vi "ImagerForFlowbit5_com.vi"() -> ()   [LabVIEW 2011]
uses:
  <vilib>/Platform/TimedLoop/XDataNode/timing_clust.ctl
  <vilib>/Platform/TimedLoop/XDataNode/nitl_modes.ctl
  <vilib>/Platform/TimedLoop/XDataNode/wakeup.ctl
  <vilib>/Instr/_visa.llb/VISA Configure Serial Port (Instr).vi
  <vilib>/Utility/config.llb/Read Key (I32).vi
  <vilib>/Analysis/1siggen.llb/Riffle Array (I32).vi
  <vilib>/Platform/TimedLoop/XDataNode/XDataNode.xnode
  <vilib>/regexp/Match Regular Expression.xnode
  <vilib>/Analysis/NI_AALBase.lvlib
  <vilib>/vision/NI_Vision_Development_Module.lvlib
  <vilib>/Platform/TimedLoop/XDataNode/XDNodeRunTimeDep.lvlib
  <vilib>/Utility/config.llb/NI_LVConfig.lvlib
panel:
  out "frameNum":i32
  out "读取缓冲区 2":string
  out "返回数 2":u32
  out "Bounds.Right":i16
  out "停止循环":bool
  in  "Stimuli":i64=5
  in  "选项卡控件":enum32{"前面板", "参数设置", "OnLineMap"}(tab)
  out "Marker":bool
  out "log":string
  out "Stim_ID":i32(listbox)=1
  in  "开始/暂停":bool=TRUE
  in  "停止":bool
  out "重排的 Stim ID":i32[](array[numeric]) caption="重排的{X}"
  out "队列中元素数量":i32
  out "Image 2":T1(plugin-control)
  in  "热图":bool
  out "循环持续时间":i64
  out "Recording":bool
  out "grabLoop":i32
  out "writeing data":bool
  out "文件编号":u32
  out "address":i16=888 caption="地址" format="%.0x"
  in  "SaveParameter":bool
  in  "Pra_binType":enum16{"Extract", "Resample"}(ring)
  in  "Pra_FramesPerStim":i64=16000
  in  "Pra_Blk目录":path=path "C:/Expt/test"
  in  "Pra_TimeForPrepare(ms)":u32=1000
  in  "Pra_stim protocol":T2(array[ring])=[enum."recording data", enum."writing data"]
  in  "Pra_blank stim":u8
  in  "Pra_wait（ms）":u32=10
  in  "Pra_ISI（ms）":u32=8000
  in  "Pra_FrameBin":i32=25
  in  "Pra_datatype":u16(ring)=13 items=["U8"=11, "I16"=12, "U32"=13, "SGL"=14]
  in  "FrameWidth":i64=704
  in  "FrameHeight":i64=576
  in  "LoadParameter":bool
  in  "Pra_bin":enum16{"1*1", "2*2"}(ring)
  in  "maker":u32[](array[numeric])
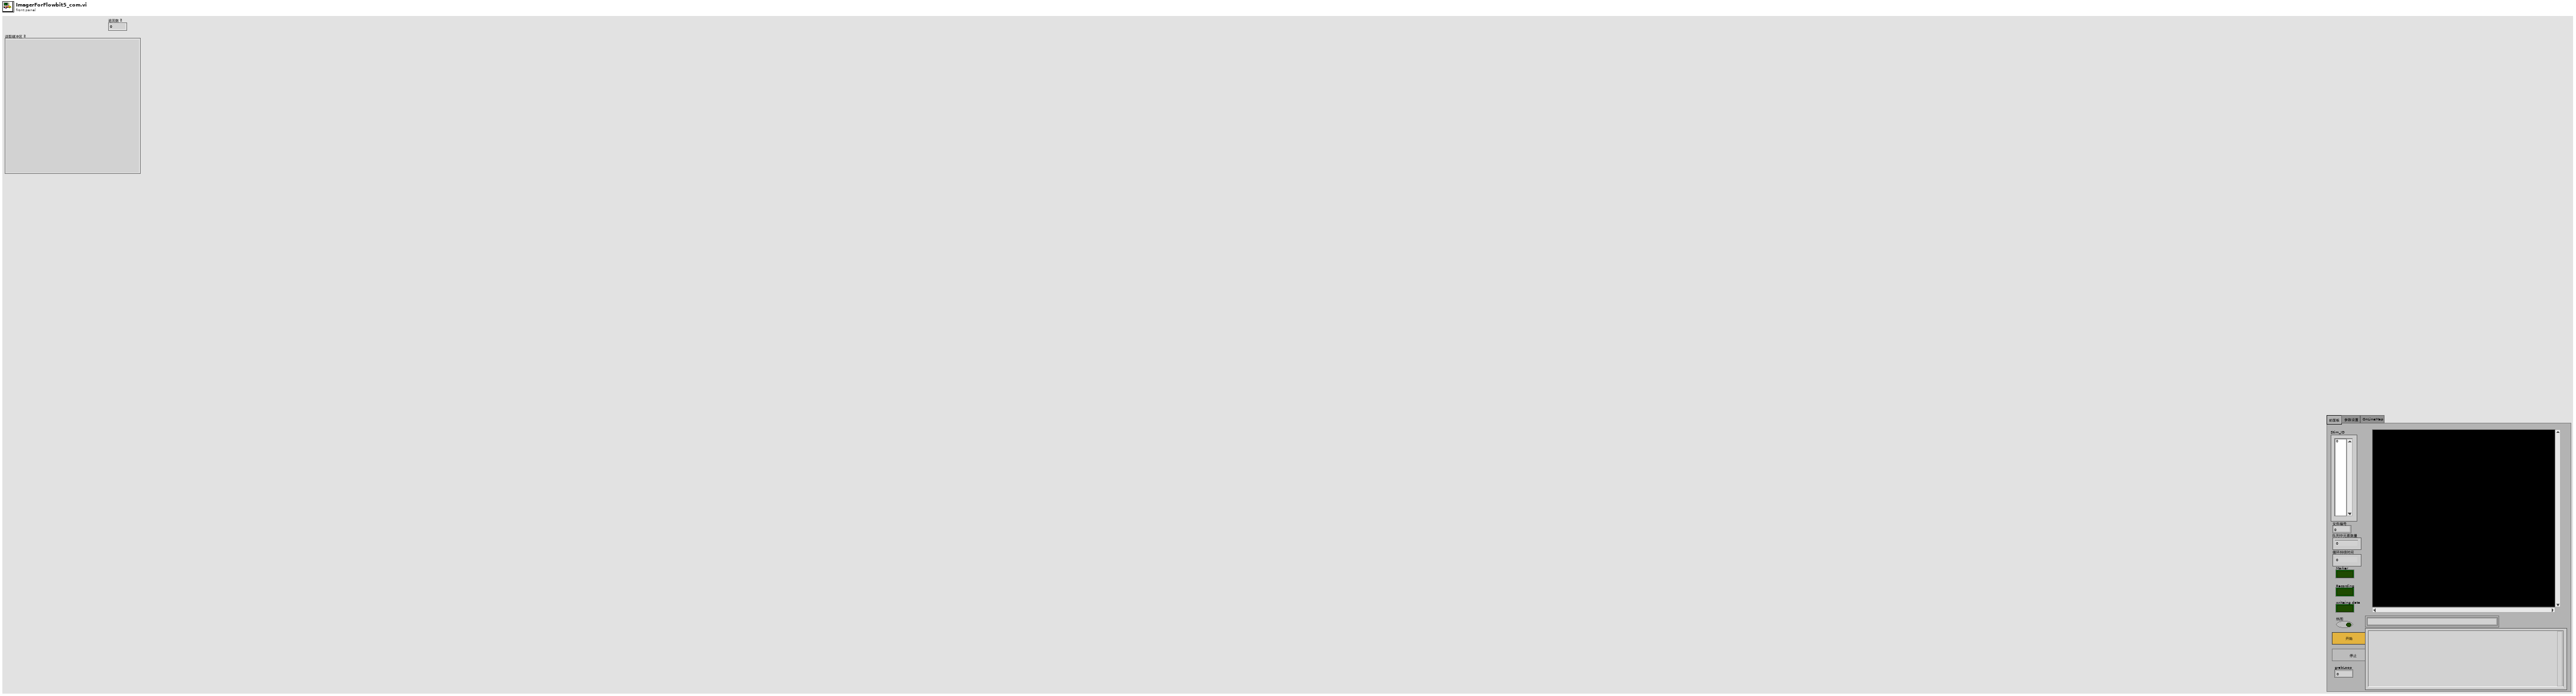
[diagram p1: front panel]
types:
  T1 = typedef "IMAQ Image.ctl" = refnum<image>
  T2 = enum16{"wait", "prep stim", "show stim", "wait respirator", "recording data", "Blank stim", "wait heart", "ISI", "DR/R", "wait calibrate", "openLightShutter", "closeLightShutter", "writing data"}[]
  T3 = typedef "Image Type" = u32
  T4 = enum16{"Disable External Trigger", "Enable External Trigger"}
  T5 = enum32{"Auto Detect", "RoadRunner", "Raven", "R64"}
  T6 = typedef "LVAllMonitorsDisplayTypeDef.ctl" = cluster{"Bounds":cluster{"Left":i16, "Top":i16, "Right":i16, "Bottom":i16}, "Depth":i16}[]
  T7 = cluster{"Bounds":cluster{"Left":i16, "Top":i16, "Right":i16, "Bottom":i16}, "Depth":i16}
  T8 = typedef "NI_LVConfig.lvlib/Config Data RefNum.ctl" = refnum<k1>
  T9 = enum16{"big-endian, network order", "native, host order", "little-endian"}
  T10 = enum16{"open", "replace", "create", "open or create", "replace or create", "replace or create with confirmation"}
  T11 = typedef "XDNodeRunTimeDep.lvlib/timing_clust.ctl" = cluster{"Expected End [f-1]":u64, "Actual End [f-1]":u64, "Finished Late? [f-1]":bool, "Expected End [i-1]":u64, "Actual End [i-1]":u64, "Finished Late? [i-1]":bool, "Expected Start [i]":u64, "Actual Start [i]":u64, "Expected Start [f]":u64, "Actual Start [f]":u64, "Source Name":string, "Structure Name":string, "Period":i64, "Deadline":i64, "Offset":i64, "Start":i64, "Priority":i32, "Timeout":i32, "Mode":T12, "Wakeup Reason":T13, "Error":errorcluster, "Source Type":string, "Secondary Source Type":string, "Global End Time":u64, "Global Start Time":u64, "Frame Duration":u64, "Iteration Duration":u64, "Assigned CPU":i32, "I/O Scan Engine Mode":u32}
  T12 = typedef "XDNodeRunTimeDep.lvlib/nitl_modes.ctl" = enum32{"No Change", "Process missed periods, maintain original phase", "Discard missed periods, maintain original phase", "Process missed periods, ignore original phase", "Discard missed periods, ignore original phase"}
  T13 = typedef "XDNodeRunTimeDep.lvlib/wakeup.ctl" = enum32{"Normal", "Aborted", "Asynchronous wakeup", "Timing source error", "Timed loop error", "Timeout"}
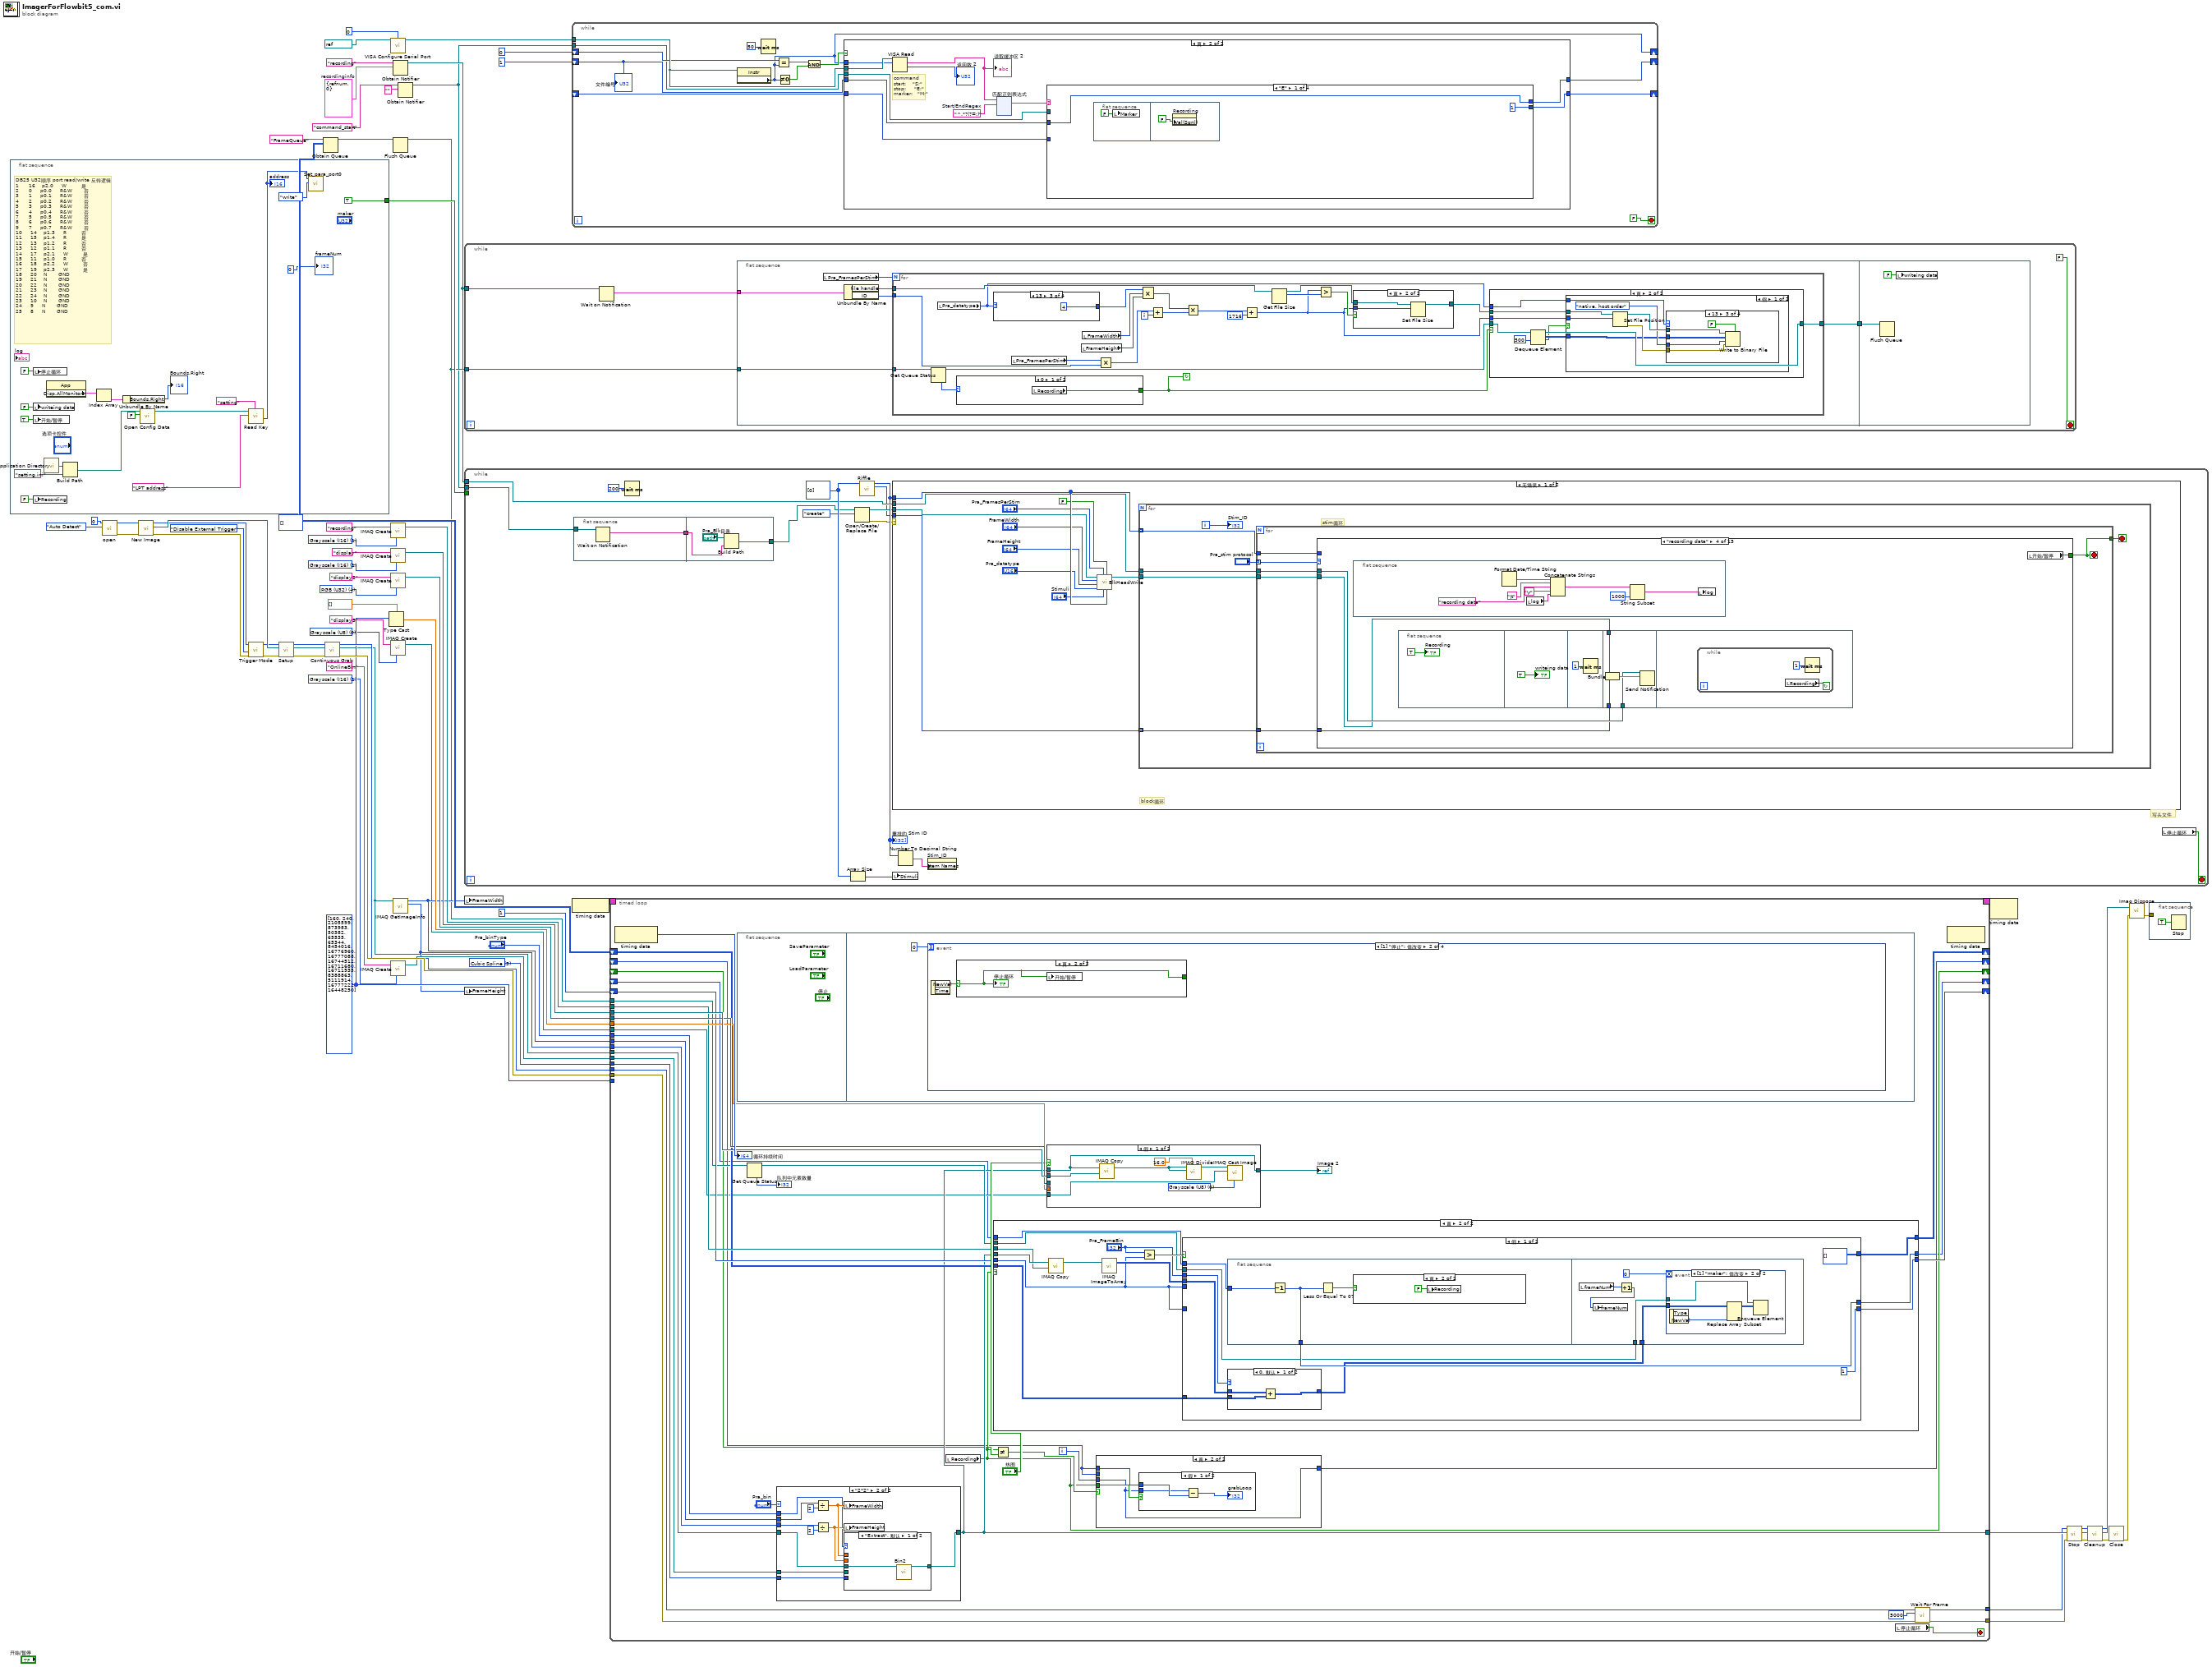
[diagram p0: block diagram]
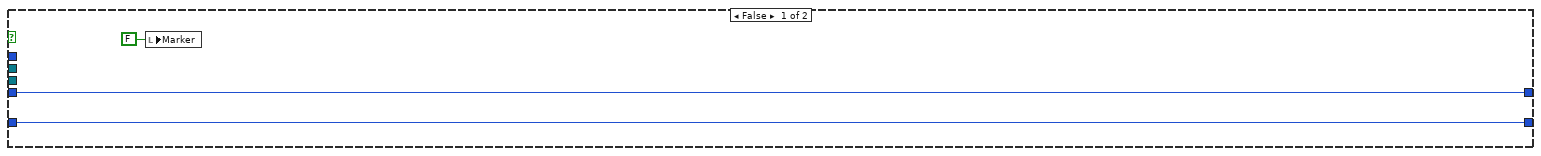
[diagram p2: hidden frame]
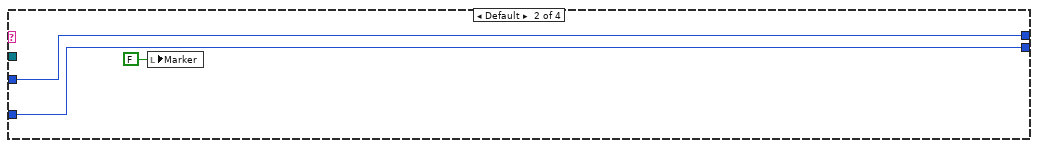
[diagram p3: hidden frame]
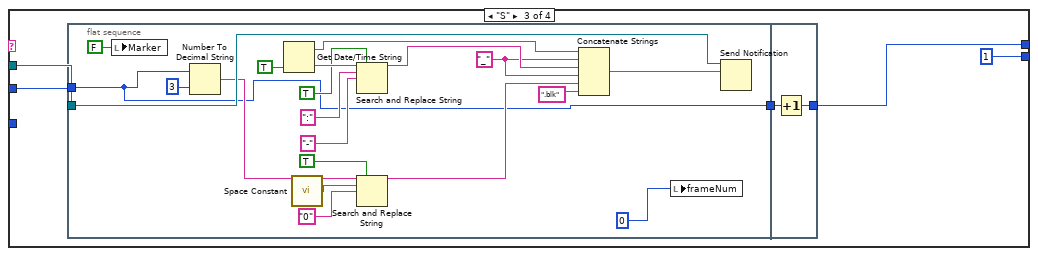
[diagram p4: hidden frame]
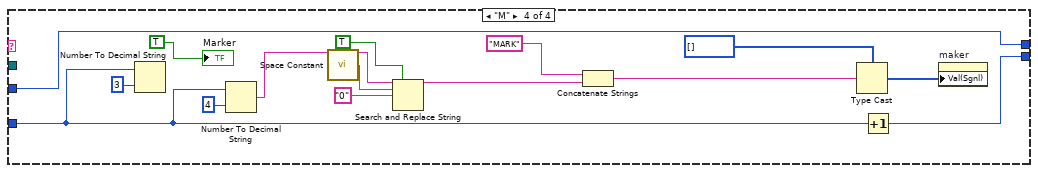
[diagram p5: hidden frame]
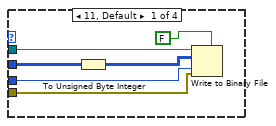
[diagram p7: hidden frame]
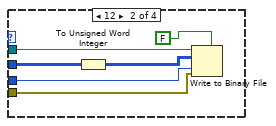
[diagram p8: hidden frame]
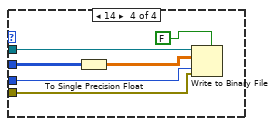
[diagram p9: hidden frame]
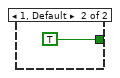
[diagram p11: hidden frame]
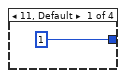
[diagram p13: hidden frame]
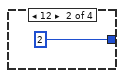
[diagram p14: hidden frame]
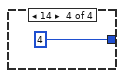
[diagram p15: hidden frame]
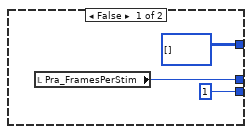
[diagram p16: hidden frame]
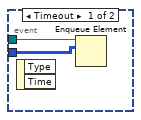
[diagram p18: hidden frame]
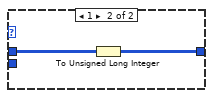
[diagram p19: hidden frame]
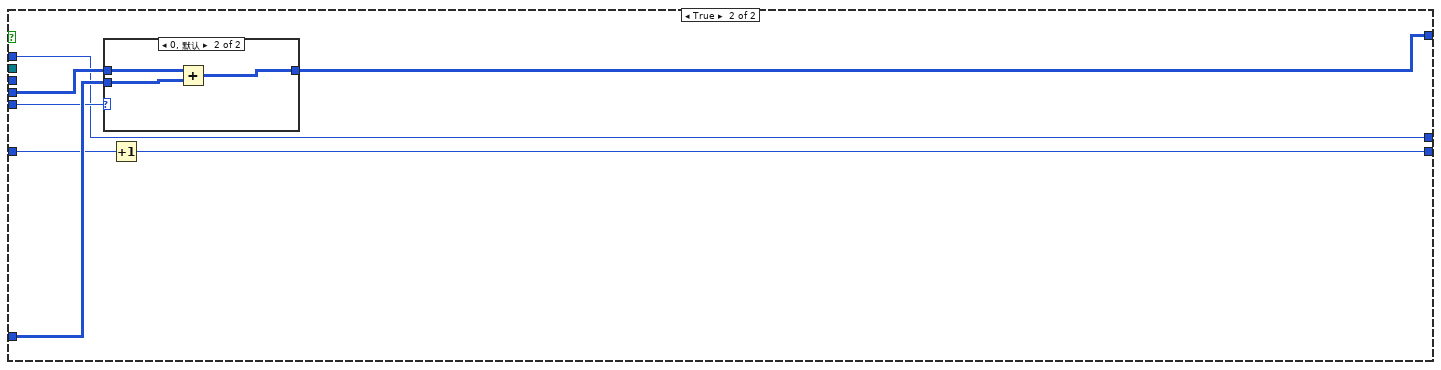
[diagram p20: hidden frame]
diagram:
  w10 = cluster{"file handle":refnum<file>, "ID":i32} {"file handle"=refnum, "ID"=0}  # recordinginfo
  w15 = T3 0 items=["Grayscale (U8)", "Grayscale (I16)", "Grayscale (SGL)", "Complex (CSG)", "RGB (U32)", "HSL (U32)", "RGB (U64)", "Grayscale (U16)"] ("Image Type")
  w20 = u32 3 items=["Zero Order", "Bi-Linear", "Quadratic", "Cubic Spline"] ("Interpolation Type")
  w22 = T3 1 items=["Grayscale (U8)", "Grayscale (I16)", "Grayscale (SGL)", "Complex (CSG)", "RGB (U32)", "HSL (U32)", "RGB (U64)", "Grayscale (U16)"] ("Image Type")
  w25 = u32[][] []
  w34 = T3 4 items=["Grayscale (U8)", "Grayscale (I16)", "Grayscale (SGL)", "Complex (CSG)", "RGB (U32)", "HSL (U32)", "RGB (U64)", "Grayscale (U16)"] ("Image Type")
  w32 = u32[] [160, 240, 2105599, 873983, 50382, 65535, 65344, 8454016, 16776960, 16777088, 16744512, 16711680, 16711935, 8388863, 5111914, 16777222, 16448250] ("数组")
  w38 = T3 1 items=["Grayscale (U8)", "Grayscale (I16)", "Grayscale (SGL)", "Complex (CSG)", "RGB (U32)", "HSL (U32)", "RGB (U64)", "Grayscale (U16)"] ("Image Type")
  w39 = T3 1 items=["Grayscale (U8)", "Grayscale (I16)", "Grayscale (SGL)", "Complex (CSG)", "RGB (U32)", "HSL (U32)", "RGB (U64)", "Grayscale (U16)"] ("Image Type")
  n1 = flat-sequence {
    tunnel: [TRUE ("Zoom to Fit Mode")] -> w27
    frame #0 {
      # "DB25\tU32顺序\tport\tread/write\t反转逻辑\n1\t     16\t   p2.0    \tW\t        是\n2\t     0    \tp0.0\t   \tR&W\t      否\n3\t     1\t\t   p0.1\t   \tR&W      \t否\n4\t\t    2\t   \tp0.2   \t\tR&W      \t否\n5\t\t    3\t\t   p0.3   \t\tR&W\t      否\n6\t\t    4\t   \tp0.4   \t\tR&W      \t否\n7\t\t    5\t   \tp0.5   \t\tR&W      \t否\n8\t\t    6\t   \tp0.6\t   \tR&W      \t否\n9\t    \t7\t   \tp0.7\t   \tR&W\t      否\n10\t    14   \tp1.3   \t\tR        \t否\n11\t   \t15   \tp1.4   \t\tR        \t是\n12\t   \t13   \tp1.2\t   \tR        \t否\n13    \t12   \tp1.1\t   \tR        \t否\n14     17   \tp2.1\t   \tW        \t是\n15    \t11   \tp1.0   \t\tR\t        否\n16    \t18   \tp2.2   \t\tW        \t否\n17    \t19\t   p2.3   \t\tW\t        是\n18    \t20   \tN   \t  \tGND\t\n19    \t21   \tN   \t  \tGND\t\n20\t    22\t   N\t  \t  \tGND\t\n21\t    23\t   N  \t  \t\tGND\t\n22\t    24\t   N  \t  \t\tGND\t\n23    \t10   \tN  \t  \t\tGND\t\n24    \t9\t    N  \t  \t\tGND\t\n25\t    8    \tN  \t  \t\tGND"
      n2 = local write "停止循环"(FALSE ("开始/暂停")) -> ()
      n3 = local write "writeing data"(FALSE ("Recording")) -> ()
      n4 = local write "开始/暂停"(TRUE ("开始/暂停")) -> ()
      n5 = local write "Recording"(FALSE ("Recording")) -> ()
      n6 = call <vilib>:"Application Directory.vi"() -> ("Application Directory"=w80:path)
      n7 = property class="App"() -> ("Disp.AllMonitors"=w72:T6)  [unwired: 2 in, 2 out]
      n8 = Build Path(base path=w80, name or relative path="setting.ini" ("名称或相对路径")) -> (appended path=w78:path)
      n9 = Index Array(array=w72) -> (element=w71:T7)  [unwired: 1 in]
      n10 = Unbundle By Name(w71) -> ("Bounds.Right"=→"Bounds.Right":i16)
      n11 = call <vilib>:"Open Config Data.vi"("create file if necessary (T)"=FALSE, "configuration file path"=w78) -> ("refnum"=w76:T8)  [unwired: 7 in, 2 out]
      n12 = call-poly <vilib>:"Read Key.vi"("section"="setting", "key"="LPT address", "refnum"=w76) -> ("value"=w73:i32)  [unwired: 5 in, 3 out]
      "address" <- w73
      n13 = call "Set_para_port0.vi"("R or W"=enum16{"read", "write"}."write", "address"=w73) -> ()  [unwired: 8 in, 2 out]
      "frameNum" <- 0
    }
  }
  n14 = call <vilib>:"open.vi"("Board Type"=T5."Auto Detect", "Board Number"=u32 0) -> ("error out"=w55:errorcluster, "RefBrdOut"=w50:u32)  [unwired: 2 in, 5 out]
  n15 = call <vilib>:"New Image.vi"("RefBrdIn"=w50, "error in"=w55) -> ("RefBrdOut"=w49:u32, "Image"=w64:T1, "error out"=w56:errorcluster)  [unwired: 6 in]
  n16 = call <vilib>:"Trigger Mode.vi"("RefBrdIn"=w49, "Trigger Mode"=T4."Disable External Trigger", "error in (no error)"=w56) -> ("RefBrdOut"=w48:u32, "error out"=w57:errorcluster)  [unwired: 6 in]
  n17 = call <vilib>:"Setup.vi"("error in"=w57, "Image In"=w64, "RefBrdIn"=w48) -> ("error out"=w52:errorcluster, "Image"=w53:T1, "RefBrdOut"=w47:u32)  [unwired: 6 in]
  n18 = Obtain Queue(name (unnamed)="FrameQueue" ("名称（未命名）"), element data type=w25) -> (queue out=w28:refnum<queue>)  [unwired: 3 in, 2 out]
  n19 = call <vilib>:"Continuous Grab.vi"("error in (no error)"=w52, "Image In"=w53, "RefBrdIn"=w47) -> ("error out"=w51:errorcluster, "Image"=w16:T1, "RefBrdOut"=w46:u32)  [unwired: 6 in]
  n20 = Type Cast(type=sgl[] [] ("单精度浮点"), x=w32) -> (*(type *) &x=w30:sgl[])
  n21 = call-poly "VISA Configure Serial Port"("VISA resource name"=refnum<visa-resource-name> "COM3", "termination char\n(0xA = '\\n' = LF)"=u8 0 ("termination char\n(0xA = '\\n' = LF)")) -> ("VISA resource name out"=w8:refnum<visa-resource-name>)  [unwired: 12 in, 1 out]
  n22 = call "IMAQ Create"("Image Name"="recording", "Image Type"=w39) -> ("New Image"=w41:T1)  [unwired: 3 in, 1 out]
  n23 = call "IMAQ Create"("Image Name"="display", "Image Type"=w38) -> ("New Image"=w36:T1)  [unwired: 3 in, 1 out]
  n24 = call "IMAQ Create"("Image Name"="display2", "Image Type"=w34) -> ("New Image"=w33:T1)  [unwired: 3 in, 1 out]
  n25 = call "IMAQ Create"("Image Name"="display3", "Image Type"=w15) -> ("New Image"=w13:T1)  [unwired: 3 in, 1 out]
  n26 = call "IMAQ Create"("Image Name"="OnlineBin", "Image Type"=w22) -> ("New Image"=w21:T1)  [unwired: 3 in, 1 out]
  n27 = Obtain Notifier(name (unnamed)="recording" ("名称（未命名）"), notification data type=w10) -> (notifier out=w9:refnum<notifier>)  [unwired: 2 in, 2 out]
  n28 = Flush Queue(queue=w28) -> (queue out=w12:refnum<queue>)  [unwired: 1 in, 2 out]
  n29 = call "IMAQ GetImageInfo"("Image"=w16) -> ("Y Resolution"=w18:i32, "X Resolution"=w19:i32)  [unwired: 3 in, 6 out]
  n30 = Obtain Notifier(name (unnamed)="command_start" ("名称（未命名）"), notification data type="" ("所有匹配")) -> (notifier out=w3:refnum<notifier>)  [unwired: 2 in, 2 out]
  n31 = while {
    tunnel: w12 -> [w90]
    tunnel: w9 -> [w89]
    stop <- FALSE stop-if-true
    n32 = Wait on Notification(notifier=w89) -> (notification=w88:cluster{"file handle":refnum<file>, "ID":i32})  [unwired: 3 in, 3 out]
    n33 = flat-sequence {
      tunnel: w90 -> [w97]
      tunnel: w88 -> [w95]
      tunnel: [w92] -> w87
      tunnel: w87 -> [w170]
      frame #0 {
        n34 = local read "Pra_FramesPerStim"() -> (w96:i64)
        n35 = Unbundle By Name(w95) -> ("file handle"=w94:refnum<file>, "ID"=w93:i32)
        n36 = for {
          N: w96 -> [_]
          tunnel: w94 -> [w120]
          tunnel: w93 -> [w110]
          tunnel: w97 -> [w101]
          tunnel: [w99] -> w92
          i -> [w108]
          stop <- w98 continue-if-true
          n37 = Get Queue Status(queue=w101) -> (queue out=w100:refnum<queue>, # elements in queue=w102:i32)  [unwired: 2 in, 6 out]
          n38 = local read "Pra_datatype"() -> (w119:u16)
          n39 = case shown="0" w102 {
            tunnel: [w160 TRUE] -> w98
            frame 0 {
              n40 = local read "Recording"() -> (w160:bool)
            }
            frame 1, Default {
            }
          }
          n41 = case shown="13" w119 {
            tunnel: [i64 1 i64 2 i64 4 i64 4] -> w114
            frame 11, Default {
            }
            frame 12 {
            }
            frame 13 {
            }
            frame 14 {
            }
          }
          n42 = local read "Pra_FramesPerStim"() -> (w111:i64)
          n43 = local read "FrameHeight"() -> (w112:i64)
          n44 = local read "FrameWidth"() -> (w113:i64)
          n45 = Multiply(x=w111, y=w110) -> (x*y=w109:i64)
          n46 = Compound Arithmetic op=MULTIPLY(w114, w113, w112) -> (w106:i64)
          n47 = Add(x=w109, y=w108) -> (x+y=w107:i64)
          n48 = Multiply(x=w106, y=w107) -> (x*y=w105:i64)
          n49 = Add(x=w105, y=i64 1716 ("x")) -> (x+y=w103:i64)
          n50 = Get File Size(file=w120) -> (refnum out=w116:refnum<file>, size (in bytes)=w115:i64)  [unwired: 1 in, 1 out]
          n51 = Greater?(x=w103, y=w115) -> (0:w117:bool)
          n52 = case shown="真" w117 {
            tunnel: w103 -> [_ w165]
            tunnel: w116 -> [w162 w164]
            tunnel: [w162 w163] -> w118
            frame False {
            }
            frame True {
              n53 = Set File Size(6:w165, 7:w164) -> (3:w163:refnum<file>)  [unwired: 1 in, 1 out]
            }
          }
          n54 = case shown="真" w98 {
            tunnel: w119 -> [_ w129]
            tunnel: w118 -> [_ w128]
            tunnel: w103 -> [_ w126]
            tunnel: w100 -> [w121 w124]
            tunnel: [w121 w123] -> w99
            frame False {
            }
            frame True {
              n55 = Dequeue Element(queue=w124, timeout in ms (-1)=500 ("超时毫秒(-1)")) -> (queue out=w123:refnum<queue>, element=w125:u32[][], timed out?=w122:bool)  [unwired: 1 in, 1 out]
              n56 = case shown="假" w122 {
                tunnel: w129 -> [w133 _]
                tunnel: w128 -> [w132 _]
                tunnel: w126 -> [w131 _]
                tunnel: w125 -> [w130 _]
                frame False {
                  n57 = Set File Position(offset (in bytes) (0)=w131, refnum=w132) -> (refnum out=w136:refnum<file>, error out=w134:errorcluster)  [unwired: 2 in]
                  n58 = case shown="13" w133 {
                    tunnel: w130 -> [w138 w145 w149 w154]
                    tunnel: w136 -> [w141 w146 w152 w156]
                    tunnel: T9."native, host order" ("字节顺序(0:big-endian, network order)") -> [w140 w147 w150 w157]
                    tunnel: w134 -> [w139 w143 w151 w158]
                    frame 11, Default {
                      n59 = To Unsigned Byte Integer(number=w138) -> (unsigned 8bit integer=w137:u8[][])
                      n60 = Write to Binary File(file (use dialog)=w141, data=w137, error in=w139, 5:FALSE ("预置数组或字符串大小？(T)"), 9:w140) -> ()  [unwired: 1 in, 3 out]
                    }
                    frame 12 {
                      n61 = To Unsigned Word Integer(number=w145) -> (unsigned 16bit integer=w144:u16[][])
                      n62 = Write to Binary File(file (use dialog)=w146, data=w144, error in=w143, 5:FALSE ("预置数组或字符串大小？(T)"), 9:w147) -> ()  [unwired: 1 in, 3 out]
                    }
                    frame 13 {
                      n63 = Write to Binary File(file (use dialog)=w152, data=w149, error in=w151, 5:FALSE ("预置数组或字符串大小？(T)"), 9:w150) -> ()  [unwired: 1 in, 3 out]
                    }
                    frame 14 {
                      n64 = To Single Precision Float(number=w154) -> (single precision float=w155:sgl[][])
                      n65 = Write to Binary File(file (use dialog)=w156, data=w155, error in=w158, 5:FALSE ("预置数组或字符串大小？(T)"), 9:w157) -> ()  [unwired: 1 in, 3 out]
                    }
                  }
                }
                frame True {
                }
              }
            }
          }
        }
      }
      frame #1 {
        n66 = Flush Queue(queue=w170) -> ()  [unwired: 1 in, 3 out]
        n67 = local write "writeing data"(FALSE ("writeing data")) -> ()
      }
    }
  }
  n68 = while {
    tunnel: w27 -> [_]
    tunnel: w9 -> [w181]
    tunnel: w3 -> [w175]
    stop <- w184 stop-if-true
    w182 = u8[] [0] ("Pra_stim ID")
    # "写头文件"
    n69 = flat-sequence {
      tunnel: w175 -> [w187]
      tunnel: [w186] -> w173
      tunnel: w173 -> [w189]
      tunnel: [w188] -> w172
      frame #0 {
        n70 = Wait on Notification(notifier=w187) -> (notification=w186:string)  [unwired: 3 in, 3 out]
      }
      frame #1 {
        n71 = Build Path(base path="Pra_Blk目录", name or relative path=w189) -> (appended path=w188:path)
      }
    }
    n72 = Wait (ms)(milliseconds to wait=u32 200 ("等待时间（毫秒）")) -> ()  [unwired: 1 out]
    n73 = Array Size(array=w182) -> (size(s)=w183:i32)
    n74 = Open/Create/Replace File(file path (use dialog)=w172, operation (0:open)=T10."create" ("操作(0:open)")) -> (refnum out=w177:refnum<file>, error out=w176:errorcluster)  [unwired: 4 in, 1 out]
    n75 = call-poly <vilib>:"Riffle.vi"("X"=w182) -> ("Riffled Index"=w174:i32[], "Riffled {X}"=w180:i32[])  [unwired: 8 in, 1 out]
    "重排的 Stim ID" <- w180
    n76 = case shown="无错误" w176 {
      tunnel: w180 -> [w200 _]
      tunnel: w174 -> [w199 _]
      tunnel: w181 -> [w198 _]
      tunnel: w177 -> [w193 _]
      frame No Error {
        # "block循环"
        n77 = call "BlkHeadWrite.vi"("SequenceOfID"=w200, "setFileSize"=FALSE, "Stimuli"="Stimuli", "FramesPerStim"="Pra_FramesPerStim", "datatype"="Pra_datatype", "FrameHeight"="FrameHeight", "FrameWidth"="FrameWidth", "引用句柄输入"=w193) -> ("引用句柄输出"=w201:refnum<file>)  [unwired: 3 in]
        n78 = for {
          tunnel: w201 -> [w208]
          tunnel: w199 -> [w207] mode=indexing
          tunnel: w200 -> [w206] mode=indexing
          tunnel: w198 -> [w202]
          i -> [w204]
          stop <- w205 stop-if-true
          # "stim循环"
          n79 = for {
            tunnel: w207 -> [w213]
            tunnel: w206 -> [w212]
            tunnel: [w210] -> w205
            tunnel: "Pra_stim protocol" -> [w211] mode=indexing
            tunnel: w208 -> [w214]
            tunnel: w202 -> [w209]
            stop <- w210 stop-if-true
            n80 = case shown="\"recording data\"" w211 {
              tunnel: w214 -> [_ _ _ w263 _ _ _ _ _ _ _ _ _]
              tunnel: w213 -> [_ _ _ w262 _ _ _ _ _ _ _ _ _]
              tunnel: w212 -> [w215 _ _ _ _ _ _ _ _ _ _ _ _]
              tunnel: [w217 w236 w250 w265 w284 w296 w309 w320 w321 w330 w331 w343 w355] -> w210
              tunnel: w209 -> [_ _ _ w264 _ _ _ _ _ _ _ _ _]
              frame "prep stim" {
                n81 = Number To Boolean Array(number=w215) -> (Boolean array=w218:bool[])
                n82 = flat-sequence {
                  tunnel: w218 -> [w229]
                  tunnel: [w229] -> w216
                  tunnel: w215 -> [w228]
                  tunnel: w216 -> [w234]
                  frame #0 {
                    n83 = Number To Decimal String(number=w228) -> (decimal integer string=w225:string)  [unwired: 1 in]
                    n84 = Format Date/Time String() -> (date/time string=w227:string)  [unwired: 3 in]
                    n85 = local read "log"() -> (w221:string)
                    n86 = Concatenate Strings(w227, "\t", "prep stim ID=" ("字符串"), w225, "\r", w221) -> (w223:string)
                    n87 = String Subset(string=w223, length (rest)=1000 ("y")) -> (substring=w222:string)  [unwired: 1 in]
                    n88 = local write "log"(w222) -> ()
                  }
                  frame #1 {
                    n89 = local read "address"() -> (w231:i16)
                    n90 = local read "address"() -> (w230:i16)
                    n91 = call "Write_para_port0.vi"("port0（8元素）"=w234, "address"=w230) -> ()  [unwired: 9 in, 1 out]
                    n92 = call "Write_para_port2_singalChange.vi"("索引"=0, "布尔"=TRUE, "address"=w231) -> ()  [unwired: 8 in, 1 out]
                  }
                  frame #2 {
                    n93 = Wait (ms)(milliseconds to wait="Pra_TimeForPrepare(ms)") -> ()  [unwired: 1 out]
                  }
                }
                n94 = local read "开始/暂停"() -> (w217:bool)
              }
              frame "wait respirator" {
                n95 = while {
                  stop <- w247 stop-if-true
                  # "this step will return true if pallel port doesn't connect any signal.That means this loop only run once."
                  n96 = Wait (ms)(milliseconds to wait=u32 5 ("等待时间（毫秒）")) -> ()  [unwired: 1 out]
                  n97 = local read "address"() -> (w245:i16)
                  n98 = call "read_para_port1.vi"("address"=w245) -> ("port1（5元素）"=w249:bool[])  [unwired: 9 in, 1 out]
                  n99 = Index Array(array=w249, index=3 ("索引")) -> (element=w247:bool)
                }
                n100 = flat-sequence {
                  frame #0 {
                    n101 = Format Date/Time String() -> (date/time string=w244:string)  [unwired: 3 in]
                    n102 = local read "log"() -> (w239:string)
                    n103 = Concatenate Strings(w244, "\t", "wait respiratory" ("字符串"), "\r", w239) -> (w241:string)
                    n104 = String Subset(string=w241, length (rest)=1000 ("y")) -> (substring=w240:string)  [unwired: 1 in]
                    n105 = local write "log"(w240) -> ()
                  }
                }
                n106 = local read "开始/暂停"() -> (w236:bool)
              }
              frame "show stim" {
                n107 = flat-sequence {
                  frame #0 {
                    n108 = local read "address"() -> (w259:i16)
                    n109 = call "Write_para_port2_singalChange.vi"("索引"=0, "布尔"=FALSE, "address"=w259) -> ()  [unwired: 8 in, 1 out]
                  }
                }
                n110 = flat-sequence {
                  frame #0 {
                    n111 = Format Date/Time String() -> (date/time string=w258:string)  [unwired: 3 in]
                    n112 = local read "log"() -> (w253:string)
                    n113 = Concatenate Strings(w258, "\t", "show stim" ("字符串"), "\r", w253) -> (w255:string)
                    n114 = String Subset(string=w255, length (rest)=1000 ("y")) -> (substring=w254:string)  [unwired: 1 in]
                    n115 = local write "log"(w254) -> ()
                  }
                }
                n116 = local read "开始/暂停"() -> (w250:bool)
              }
              frame "recording data" {
                n117 = flat-sequence {
                  frame #0 {
                    n118 = Format Date/Time String() -> (date/time string=w282:string)  [unwired: 3 in]
                    n119 = local read "log"() -> (w277:string)
                    n120 = Concatenate Strings(w282, "\t", "recording data" ("字符串"), "\r", w277) -> (w279:string)
                    n121 = String Subset(string=w279, length (rest)=1000 ("y")) -> (substring=w278:string)  [unwired: 1 in]
                    n122 = local write "log"(w278) -> ()
                  }
                }
                n123 = flat-sequence {
                  tunnel: w264 -> [w271]
                  tunnel: w263 -> [w270]
                  tunnel: w262 -> [w269]
                  frame #0 {
                    "Recording" <- TRUE ("Recording")
                  }
                  frame #1 {
                    "writeing data" <- TRUE ("Recording")
                  }
                  frame #2 {
                    n124 = Wait (ms)(milliseconds to wait=u32 1 ("等待时间（毫秒）")) -> ()  [unwired: 1 out]
                  }
                  frame #3 {
                    n125 = Bundle("引用句柄输出"=w270, w269) -> (w272:cluster{"引用句柄输出":refnum<file>, i32})  [unwired: 1 in]
                    n126 = Send Notification(notification=w272, notifier=w271) -> ()  [unwired: 1 in, 2 out]
                  }
                  frame #4 {
                    n127 = while {
                      stop <- w274 continue-if-true
                      n128 = local read "Recording"() -> (w274:bool)
                      n129 = Wait (ms)(milliseconds to wait=u32 1 ("等待时间（毫秒）")) -> ()  [unwired: 1 out]
                    }
                  }
                }
                n130 = local read "开始/暂停"() -> (w265:bool)
              }
              frame "Blank stim" {
                n131 = flat-sequence {
                  frame #0 {
                    n132 = Format Date/Time String() -> (date/time string=w294:string)  [unwired: 3 in]
                    n133 = local read "log"() -> (w289:string)
                    n134 = Concatenate Strings(w294, "\t", "show blank stim" ("字符串"), "\r", w289) -> (w291:string)
                    n135 = String Subset(string=w291, length (rest)=1000 ("y")) -> (substring=w290:string)  [unwired: 1 in]
                    n136 = local write "log"(w290) -> ()
                  }
                }
                n137 = local read "address"() -> (w283:i16)
                n138 = Number To Boolean Array(number="Pra_blank stim") -> (Boolean array=w285:bool[])
                n139 = call "Write_para_port0.vi"("port0（8元素）"=w285, "address"=w283) -> ()  [unwired: 9 in, 1 out]
                n140 = local read "开始/暂停"() -> (w284:bool)
              }
              frame "ISI" {
                n141 = flat-sequence {
                  tunnel: "Pra_ISI（ms）" -> [w300]
                  tunnel: "Pra_ISI（ms）" -> [w307]
                  frame #0 {
                    n142 = Number To Decimal String(number=w300) -> (decimal integer string=w304:string)  [unwired: 1 in]
                    n143 = Format Date/Time String() -> (date/time string=w306:string)  [unwired: 3 in]
                    n144 = local read "log"() -> (w299:string)
                    n145 = Concatenate Strings(w306, "\t", "ISI(ms)=" ("字符串"), w304, "\r", w299) -> (w302:string)
                    n146 = String Subset(string=w302, length (rest)=1000 ("y")) -> (substring=w301:string)  [unwired: 1 in]
                    n147 = local write "log"(w301) -> ()
                  }
                  frame #1 {
                    n148 = Wait (ms)(milliseconds to wait=w307) -> ()  [unwired: 1 out]
                  }
                }
                n149 = local read "开始/暂停"() -> (w296:bool)
              }
              frame "wait", Default {
                n150 = Wait (ms)(milliseconds to wait="Pra_wait（ms）") -> ()  [unwired: 1 out]
                n151 = flat-sequence {
                  tunnel: "Pra_wait（ms）" -> [w313]
                  frame #0 {
                    n152 = Number To Decimal String(number=w313) -> (decimal integer string=w317:string)  [unwired: 1 in]
                    n153 = Format Date/Time String() -> (date/time string=w319:string)  [unwired: 3 in]
                    n154 = local read "log"() -> (w312:string)
                    n155 = Concatenate Strings(w319, "\t", "wait(ms)=" ("字符串"), w317, "\r", w312) -> (w315:string)
                    n156 = String Subset(string=w315, length (rest)=1000 ("y")) -> (substring=w314:string)  [unwired: 1 in]
                    n157 = local write "log"(w314) -> ()
                  }
                }
                n158 = local read "开始/暂停"() -> (w309:bool)
              }
              frame "DR/R" {
                n159 = local read "开始/暂停"() -> (w320:bool)
              }
              frame "wait heart" {
                n160 = flat-sequence {
                  frame #0 {
                    n161 = Format Date/Time String() -> (date/time string=w329:string)  [unwired: 3 in]
                    n162 = local read "log"() -> (w324:string)
                    n163 = Concatenate Strings(w329, "\t", "wait heart" ("字符串"), "\r", w324) -> (w326:string)
                    n164 = String Subset(string=w326, length (rest)=1000 ("y")) -> (substring=w325:string)  [unwired: 1 in]
                    n165 = local write "log"(w325) -> ()
                  }
                }
                n166 = local read "开始/暂停"() -> (w321:bool)
              }
              frame "wait calibrate" {
                n167 = local read "开始/暂停"() -> (w330:bool)
              }
              frame "openLightShutter" {
                n168 = flat-sequence {
                  frame #0 {
                    n169 = local read "address"() -> (w340:i16)
                    n170 = call "Write_para_port2_singalChange.vi"("索引"=1, "布尔"=TRUE, "address"=w340) -> ()  [unwired: 8 in, 1 out]
                  }
                }
                n171 = flat-sequence {
                  frame #0 {
                    n172 = Format Date/Time String() -> (date/time string=w339:string)  [unwired: 3 in]
                    n173 = local read "log"() -> (w334:string)
                    n174 = Concatenate Strings(w339, "\t", "open light shutter" ("字符串"), "\r", w334) -> (w336:string)
                    n175 = String Subset(string=w336, length (rest)=1000 ("y")) -> (substring=w335:string)  [unwired: 1 in]
                    n176 = local write "log"(w335) -> ()
                  }
                }
                n177 = local read "开始/暂停"() -> (w331:bool)
              }
              frame "closeLightShutter" {
                n178 = flat-sequence {
                  frame #0 {
                    n179 = local read "address"() -> (w352:i16)
                    n180 = call "Write_para_port2_singalChange.vi"("索引"=1, "布尔"=FALSE, "address"=w352) -> ()  [unwired: 8 in, 1 out]
                  }
                }
                n181 = flat-sequence {
                  frame #0 {
                    n182 = Format Date/Time String() -> (date/time string=w351:string)  [unwired: 3 in]
                    n183 = local read "log"() -> (w346:string)
                    n184 = Concatenate Strings(w351, "\t", "close light shutter" ("字符串"), "\r", w346) -> (w348:string)
                    n185 = String Subset(string=w348, length (rest)=1000 ("y")) -> (substring=w347:string)  [unwired: 1 in]
                    n186 = local write "log"(w347) -> ()
                  }
                }
                n187 = local read "开始/暂停"() -> (w343:bool)
              }
              frame "writing data" {
                n188 = while {
                  stop <- w364 continue-if-true
                  n189 = local read "writeing data"() -> (w364:bool)
                  n190 = Wait (ms)(milliseconds to wait=u32 1 ("等待时间（毫秒）")) -> ()  [unwired: 1 out]
                }
                n191 = flat-sequence {
                  frame #0 {
                    n192 = Format Date/Time String() -> (date/time string=w363:string)  [unwired: 3 in]
                    n193 = local read "log"() -> (w358:string)
                    n194 = Concatenate Strings(w363, "\t", "writing data" ("字符串"), "\r", w358) -> (w360:string)
                    n195 = String Subset(string=w360, length (rest)=1000 ("y")) -> (substring=w359:string)  [unwired: 1 in]
                    n196 = local write "log"(w359) -> ()
                  }
                }
                n197 = local read "开始/暂停"() -> (w355:bool)
              }
            }
          }
          "Stim_ID" <- w204
        }
      }
      frame Error {
        (unwired) TRUE ("开始/暂停")
        n198 = local write "开始/暂停"(TRUE ("开始/暂停")) -> ()
        n199 = One Button Dialog(message="blk exist, please change the file name" ("消息")) -> ()  [unwired: 1 in, 1 out]
      }
    }
    n200 = local write "Stimuli"(w183) -> ()
    n201 = Number To Decimal String(number=w180) -> (decimal integer string=w179:string[])  [unwired: 1 in]
    n202 = property on="Stim_ID" class="LstBox (严格)"("Item Names"=w179) -> ()  [unwired: 2 in, 2 out]
    n203 = local read "停止循环"() -> (w184:bool)
  }
  n204 = local write "FrameWidth"(w19) -> ()
  n205 = local write "FrameHeight"(w18) -> ()
  n206 = while {
    tunnel: w8 -> [w379]
    shift-right: [w373] -> _
    shift-left: u32 0 ("Bytes at Port") -> [w377]
    tunnel: w3 -> [w372]
    shift-right: [w371] -> _
    shift-left: _ -> [w370]
    shift-right: [w368] -> _
    shift-left: u32 1 ("Bytes at Port") -> [w369]
    stop <- FALSE stop-if-true
    n207 = property class="Instr"(reference=w379) -> ("Serial Settings:Number of Bytes at Serial Port"=w373:u32)  [unwired: 1 in, 2 out]
    n208 = Wait (ms)(milliseconds to wait=u32 50 ("等待时间（毫秒）")) -> ()  [unwired: 1 out]
    n209 = Equal?(x=w377, y=w373) -> (x = y?=w376:bool)
    n210 = Not Equal To 0?(x=w373) -> (x != 0?=w375:bool)
    n211 = And(x=w376, y=w375) -> (x .and. y?=w374:bool)
    n212 = case shown="真" w374 {
      tunnel: w379 -> [_ w393]
      tunnel: w373 -> [_ w392]
      tunnel: w372 -> [_ w388]
      tunnel: [w383 w387] -> w371
      tunnel: w370 -> [w383 w386]
      tunnel: w369 -> [w382 w385]
      tunnel: [w382 w384] -> w368
      frame False {
        n213 = local write "Marker"(FALSE ("Maker")) -> ()
      }
      frame True {
        w391 = "^.*?(?=;)"  # Start/EndRegex
        # "command\nstart:    \"S;\"\nstop:     \"E;\"\nmarker:   \"M;\""
        n214 = VISA Read(VISA resource name=w393, byte count=w392) -> (read buffer=w389:string, return count=→"返回数 2":u32)  [unwired: 1 in, 2 out]
        "读取缓冲区 2" <- w389
        n215 = xnode "匹配正则表达式"("输入字符串"=w389, "正则表达式"=w391) -> ("所有匹配"=w390:string)  [unwired: 4 in, 4 out]
        n216 = case shown="\"E\"" w390 {
          tunnel: w388 -> [_ _ w406 _]
          tunnel: [1 w401 1 w443] -> w387
          tunnel: w386 -> [_ w401 _ w436]
          tunnel: w385 -> [w395 w400 w404 w430]
          tunnel: [w395 w400 w403 w430] -> w384
          frame "E" {
            n217 = flat-sequence {
              frame #0 {
                n218 = local write "Marker"(FALSE ("Maker")) -> ()
              }
              frame #1 {
                n219 = property on="Recording" class="Bool (严格)"("Val(Sgnl)"=FALSE ("Recording")) -> ()  [unwired: 2 in, 2 out]
              }
            }
          }
          frame Default {
            n220 = local write "Marker"(FALSE ("Maker")) -> ()
          }
          frame "S" {
            n221 = flat-sequence {
              tunnel: w406 -> [w426]
              tunnel: w404 -> [w407]
              tunnel: [w407] -> w402
              tunnel: [w428] -> w403
              tunnel: w402 -> [w427]
              frame #0 {
                w413 = "_" ("字符串")
                n222 = local write "Marker"(FALSE ("Maker")) -> ()
                n223 = Number To Decimal String(number=w407, width (-)=i16 3 ("宽度(-)")) -> (decimal integer string=w422:string)
                n224 = Get Date/Time String(want seconds? (F)=TRUE ("需要秒？(F)")) -> (date string=w419:string, time string=w418:string)  [unwired: 2 in]
                n225 = call <vilib>:"Space Constant.vi"() -> ("String"=w424:string)
                n226 = Search and Replace String(replace all?=TRUE ("替换全部？(F)"), input string=w418, search string=":" ("搜索字符串"), replace string="-" ("替换字符串(\"\")")) -> (result string=w414:string)  [unwired: 4 in, 3 out]
                n227 = Search and Replace String(replace all?=TRUE ("替换全部？(F)"), input string=w422, search string=w424, replace string="0" ("替换字符串(\"\")")) -> (result string=w412:string)  [unwired: 4 in, 3 out]
                n228 = Concatenate Strings(w419, w413, w414, w413, w412, ".blk" ("字符串")) -> (w411:string)
                n229 = local write "frameNum"(0 ("frameNum")) -> ()
                n230 = Send Notification(notification=w411, notifier=w426) -> ()  [unwired: 1 in, 2 out]
              }
              frame #1 {
                n231 = Increment(x=w427) -> (x+1=w428:u32)
              }
            }
          }
          frame "M" {
            n232 = Number To Decimal String(number=w436, width (-)=i16 3 ("宽度(-)")) -> ()  [unwired: 1 out]
            n233 = Number To Decimal String(number=w436, width (-)=i16 4 ("宽度(-)")) -> (decimal integer string=w440:string)
            n234 = call <vilib>:"Space Constant.vi"() -> ("String"=w439:string)
            n235 = Search and Replace String(replace all?=TRUE ("替换全部？(F)"), input string=w440, search string=w439, replace string="0" ("替换字符串(\"\")")) -> (result string=w434:string)  [unwired: 4 in, 3 out]
            n236 = Concatenate Strings("MARK", w434) -> (w431:string)
            n237 = Type Cast(type=u32[] [], x=w431) -> (*(type *) &x=w432:u32[])
            n238 = Increment(x=w436) -> (x+1=w443:i32)
            n239 = property on="maker" class="Arr (严格)"("Val(Sgnl)"=w432) -> ()  [unwired: 2 in, 2 out]
            "Marker" <- TRUE ("Maker")
          }
        }
      }
    }
    "文件编号" <- w369
  }
  n240 = node-c288() -> (w68:T11)
  n241 = timed-loop {
    tunnel: [w569] -> w63
    tunnel: [w591] -> w58
    tunnel: w16 -> [w570]
    tunnel: w51 -> [w590]
    tunnel: w46 -> [w589]
    tunnel: [w588] -> w45
    timing: w68 -> [_]
    timing-out: [_] -> w67
    tunnel: w41 -> [w579]
    tunnel: w12 -> [w574]
    tunnel: w36 -> [w584]
    tunnel: w32 -> [_]
    tunnel: w33 -> [w583]
    tunnel: w30 -> [w582]
    shift-right: [w577] -> _
    shift-left: 1 -> [w578]
    shift-right: [w576] -> _
    shift-left: w25 -> [w575]
    tunnel: w21 -> [w572]
    tunnel: w20 -> [w571]
    tunnel: w19 -> [w567]
    tunnel: w18 -> [w566]
    tunnel: "Pra_binType" -> [w565]
    shift-right: [w559] -> _
    shift-left: _ -> [w563]
    shift-right: [w560] -> _
    shift-left: _ -> [w558]
    tunnel: w13 -> [w557]
    shift-right: [w556] -> _
    shift-left: _ -> [w555]
    i -> [w561]
    stop <- w585 stop-if-true
    n242 = node-c288() -> (→"循环持续时间":i64)  [unwired: 1 in]
    n243 = flat-sequence {
      frame #0 {
      }
      frame #1 {
        n244 = event shown="[1] \"停止\": 值改变" {
          selector: _ -> [_ _ _ _]
          dyn-events: _ -> [_ _ _ _]
          timeout: 0 -> [_ _ _ _]
          event Timeout {
            n245 = event-data() -> ()  [unwired: 1 in, 2 out]
          }
          event "停止": Value Change {
            n246 = event-data() -> ("NewVal"=w676:bool)  [unwired: 1 in, 1 out]
            n247 = case shown="真" w676 {
              selector: w676 -> [_ w678]
              tunnel: [FALSE w678] -> _
              frame False {
              }
              frame True {
                n248 = local write "开始/暂停"(w678) -> ()
                "停止循环" <- w678
              }
            }
          }
          event "SaveParameter": Value Change {
            n249 = event-data() -> ()  [unwired: 1 in, 1 out]
            n250 = call "文件对话框"("prompt"="SaveParameterTo", "pattern (all files)"="*.prmf", "pattern label"="Flowbit") -> ("selected path"=w680:path, "error out"=w682:errorcluster)  [unwired: 9 in, 2 out]
            n251 = case shown="无错误" w682 {
              tunnel: w680 -> [w685 _]
              frame No Error {
                n252 = control-ref of="本VI"() -> (w689:refnum<vi>)
                n253 = invoke class="VI" method="Ctrl Val.Get All"(reference=w689, "Controls"=TRUE ("输入控件")) -> ("Get All Control Values Variant"=w688:cluster{"Name":string, "Variant Data":variant}[])  [unwired: 2 in, 3 out]
                n254 = for {
                  tunnel: w688 -> [w693] mode=indexing
                  shift-right: [w692] -> w686
                  shift-left: cluster{"Name":string, "Variant Data":variant}[] [] -> [w691]
                  i -> [w690]
                  n255 = Unbundle By Name(w693) -> ("Name"=w698:string)
                  n256 = String Subset(string=w698, length (rest)=4 ("长度（剩余）")) -> (substring=w696:string)  [unwired: 1 in]
                  n257 = Equal?(x=w696, y="Pra_") -> (x = y?=w694:bool)
                  n258 = case shown="真" w694 {
                    tunnel: w693 -> [_ w703]
                    tunnel: [w699 w702] -> w692
                    tunnel: w691 -> [w699 w701]
                    tunnel: w690 -> [_ w700]
                    frame False {
                    }
                    frame True {
                      n259 = case shown="0" w700 {
                        tunnel: w703 -> [w705 w708]
                        tunnel: [w704 w707] -> w702
                        tunnel: w701 -> [_ w706]
                        frame 0 {
                          n260 = Build Array(w705) -> (w704:cluster{"Name":string, "Variant Data":variant}[])
                        }
                        frame 1, Default {
                          n261 = Build Array (concatenate)(w706, w708) -> (w707:cluster{"Name":string, "Variant Data":variant}[])
                        }
                      }
                    }
                  }
                }
                n262 = Write to Binary File(file (use dialog)=w685, data=w686) -> ()  [unwired: 4 in, 3 out]
              }
              frame Error {
              }
            }
          }
          event "LoadParameter": Value Change {
            n263 = event-data() -> ()  [unwired: 1 in, 1 out]
            n264 = call "文件对话框2"("prompt"="LoadParameter", "pattern (all files)"="*.prmf", "pattern label"="Flowbit") -> ("selected path"=w709:path, "error out"=w710:errorcluster)  [unwired: 9 in, 2 out]
            n265 = case shown="无错误" w710 {
              tunnel: w709 -> [w717 _]
              frame No Error {
                n266 = Read from Binary File(5:cluster{"Name":string, "Variant Data":variant}[] [], 11:w717) -> (2:w714:cluster{"Name":string, "Variant Data":variant}[])  [unwired: 4 in, 3 out]
                n267 = control-ref of="本VI"() -> (w715:refnum<vi>)
                n268 = for {
                  tunnel: w715 -> [w722]
                  tunnel: w714 -> [w721] mode=indexing
                  n269 = Unbundle By Name(w721) -> ("Name"=w720:string, "Variant Data"=w719:variant)
                  n270 = invoke class="VI" method="Ctrl Val.Set"(reference=w722, "Control Name"=w720, "Value"=w719) -> (error out=w718:errorcluster)  [unwired: 2 in, 4 out]
                  n271 = call <vilib>:"Clear Errors.vi"("error in (no error)"=w718) -> ()  [unwired: 6 in, 1 out]
                }
              }
              frame Error {
              }
            }
          }
        }
      }
    }
    n272 = Get Queue Status(queue=w574) -> (queue out=w573:refnum<queue>, # elements in queue=→"队列中元素数量":i32)  [unwired: 2 in, 6 out]
    n273 = case shown="\"2*2\"" "Pra_bin" {
      tunnel: w572 -> [_ w662]
      tunnel: w571 -> [_ w657]
      tunnel: w570 -> [w655 w661]
      tunnel: [w655 w660] -> w569
      tunnel: w567 -> [_ w666]
      tunnel: w566 -> [_ w663]
      tunnel: w565 -> [_ w656]
      frame "1*1", Default {
      }
      frame "2*2" {
        n274 = Divide(x=w666, y=2) -> (x/y=w659:dbl)
        n275 = Divide(x=w663, y=2) -> (x/y=w658:dbl)
        n276 = local write "FrameWidth"(w659) -> ()
        n277 = local write "FrameHeight"(w658) -> ()
        n278 = case shown="\"Extract\", 默认" w656 {
          tunnel: w662 -> [_ w673]
          tunnel: w661 -> [w668 w674]
          tunnel: [w667 w670] -> w660
          tunnel: w659 -> [_ w672]
          tunnel: w658 -> [_ w671]
          tunnel: w657 -> [_ w669]
          frame "Extract", Default {
            n279 = call "Bin2.vi"("Image Src"=w668) -> ("Image"=w667:T1)  [unwired: 10 in]
          }
          frame "Resample" {
            n280 = call "IMAQ Resample"("X Resolution"=w672, "Y Resolution"=w671, "Interpolation Type"=w669, "Image Dst"=w673, "Image Src"=w674) -> ("Image Dst Out"=w670:T1)  [unwired: 5 in, 1 out]
          }
        }
      }
    }
    n281 = local read "Recording"() -> (w559:bool)
    n282 = case shown="真" w559 {
      tunnel: w573 -> [_ w602]
      tunnel: w569 -> [_ w607]
      tunnel: w579 -> [_ w606]
      tunnel: w578 -> [_ w598]
      tunnel: [1 w603] -> w577
      tunnel: w575 -> [_ w599]
      tunnel: [u32[][] [] w601] -> w576
      tunnel: [w592 w595] -> w556
      tunnel: w555 -> [_ w596]
      frame False {
        n283 = local read "Pra_FramesPerStim"() -> (w592:i64)
      }
      frame True {
        n284 = call "IMAQ Copy"("Image Dst"=w606, "Image Src"=w607) -> ("Image Dst Out"=w605:T1)  [unwired: 4 in, 1 out]
        n285 = call "IMAQ ImageToArray"("Image"=w605) -> ("Image Pixels (I16)"=w600:i16[][])  [unwired: 3 in, 4 out]
        n286 = Greater?(x="Pra_FrameBin", y=w598) -> (0:w604:bool)
        n287 = case shown="假" w604 {
          tunnel: w598 -> [_ w639]
          tunnel: [1 w638] -> w603
          tunnel: w602 -> [w609 _]
          tunnel: [u32[][] [] w641] -> w601
          tunnel: w600 -> [w615 w643]
          tunnel: w599 -> [w614 w642]
          tunnel: w598 -> [_ w640]
          tunnel: "Pra_FrameBin" -> [w612 _]
          tunnel: w596 -> [w611 w637]
          tunnel: [w610 w637] -> w595
          frame False {
            n288 = flat-sequence {
              tunnel: w611 -> [w619]
              tunnel: [w617] -> w610
              tunnel: w609 -> [w625]
              tunnel: w608 -> [w624]
              frame #0 {
                n289 = Decrement(x=w619) -> (x-1=w617:i64)
                n290 = Less Or Equal To 0?(x=w617) -> (x <= 0?=w618:bool)
                n291 = case shown="真" w618 {
                  frame False {
                  }
                  frame True {
                    n292 = local write "Recording"(FALSE ("Recording")) -> ()
                  }
                }
              }
              frame #1 {
                n293 = local read "frameNum"() -> (w622:i32)
                n294 = Increment(x=w622) -> (x+1=w621:i32)
                n295 = local write "frameNum"(w621) -> ()
                n296 = event shown="[1] \"maker\": 值改变" {
                  selector: _ -> [_ _]
                  dyn-events: _ -> [_ _]
                  timeout: 0 -> [_ _]
                  tunnel: w625 -> [w627 w631]
                  tunnel: w624 -> [w626 w630]
                  event Timeout {
                    n297 = event-data() -> ()  [unwired: 1 in, 2 out]
                    n298 = Enqueue Element(queue=w627, element=w626) -> ()  [unwired: 2 in, 3 out]
                  }
                  event "maker": Value Change {
                    n299 = event-data() -> ("NewVal"=w629:u32[])  [unwired: 1 in, 1 out]
                    n300 = Replace Array Subset(array=w630, new element=w629) -> (w628:u32[][])  [unwired: 2 in]
                    n301 = Enqueue Element(queue=w631, element=w628) -> ()  [unwired: 2 in, 3 out]
                  }
                }
              }
            }
            n302 = case shown="0, 默认" w612 {
              tunnel: w615 -> [w634 w636]
              tunnel: w614 -> [w633 _]
              tunnel: [w632 w635] -> w608
              frame 0, Default {
                n303 = Add(x=w634, y=w633) -> (x+y=w632:u32[][])
              }
              frame 1 {
                n304 = To Unsigned Long Integer(number=w636) -> (unsigned 32bit integer=w635:u32[][])
              }
            }
          }
          frame True {
            n305 = case shown="0, 默认" w640 {
              tunnel: w643 -> [w644 w647]
              tunnel: w642 -> [_ w646]
              tunnel: [w644 w645] -> w641
              frame 1 {
              }
              frame 0, Default {
                n306 = Add(x=w647, y=w646) -> (x+y=w645:u32[][])
              }
            }
            n307 = Increment(x=w639) -> (x+1=w638:i32)
          }
        }
      }
    }
    n308 = Not Equal?(x=w559, y=w563) -> (x != y?=w562:bool)
    n309 = case shown="假" "热图" {
      tunnel: w584 -> [w729 w737]
      tunnel: w569 -> [w723 w735]
      tunnel: [w723 w734] -> w581
      tunnel: w583 -> [_ w732]
      tunnel: w582 -> [_ w731]
      tunnel: w557 -> [w727 _]
      frame False {
        w728 = T3 0 items=["Grayscale (U8)", "Grayscale (I16)", "Grayscale (SGL)", "Complex (CSG)", "RGB (U32)", "HSL (U32)", "RGB (U64)", "Grayscale (U16)"] ("Image Type")
        n310 = call "IMAQ Copy"("Image Dst"=w729, "Image Src"=w723) -> ("Image Dst Out"=w726:T1)  [unwired: 4 in, 1 out]
        n311 = call "IMAQ Divide"("Image Src A"=w726, "Constant"=sgl 16.0, "Image Dst"=w726) -> ("Image Dst Out"=w724:T1)  [unwired: 4 in, 1 out]
        n312 = call "IMAQ Cast Image"("Image Type"=w728, "Image Dst"=w727, "Image Src"=w724) -> ()  [unwired: 7 in, 2 out]
      }
      frame True {
        w733 = T3 4 items=["Grayscale (U8)", "Grayscale (I16)", "Grayscale (SGL)", "Complex (CSG)", "RGB (U32)", "HSL (U32)", "RGB (U64)", "Grayscale (U16)"] ("Image Type")
        n313 = call "IMAQ Copy"("Image Dst"=w737, "Image Src"=w735) -> ("Image Dst Out"=w736:T1)  [unwired: 4 in, 1 out]
        n314 = call "IMAQ Divide"("Image Src A"=w736, "Constant"=sgl 256.0, "Image Dst"=w736) -> ("Image Dst Out"=w730:T1)  [unwired: 4 in, 1 out]
        n315 = call "IMAQ Cast Image"("Image Type"=w733, "Lookup Table"=w731, "Image Dst"=w732, "Image Src"=w730) -> ("Image Dst Out"=w734:T1)  [unwired: 6 in, 1 out]
      }
    }
    "Image 2" <- w581
    n316 = case shown="真" w562 {
      tunnel: w561 -> [_ w649]
      tunnel: [w648 w649] -> w560
      tunnel: w558 -> [w648 w650]
      tunnel: w559 -> [_ w651]
      tunnel: w558 -> [_ _]
      frame False {
      }
      frame True {
        n317 = case shown="假" w651 {
          tunnel: w650 -> [w653 _]
          tunnel: w649 -> [w652 _]
          frame False {
            n318 = Subtract(x=w652, y=w653) -> (x-y=→"grabLoop":i32)
          }
          frame True {
          }
        }
      }
    }
    n319 = local read "停止循环"() -> (w585:bool)
    n320 = call <vilib>:"Wait For Frame.vi"("error in (no error)"=w590, "Timeout (mS)"=u32 5000, "RefBrdIn"=w589) -> ("error out"=w591:errorcluster, "RefBrdOut"=w588:u32)  [unwired: 7 in]
    n321 = node-c288() -> ()  [unwired: 1 in, 1 out]
  }
  n322 = node-c288(w67) -> ()  [unwired: 1 out]
  n323 = call <vilib>:"Stop.vi"("error in (no error)"=w58, "Image In"=w63, "RefBrdIn"=w45) -> ("error out"=w59:errorcluster, "Image"=w62:T1, "RefBrdOut"=w44:u32)  [unwired: 6 in]
  n324 = call <vilib>:"Cleanup.vi"("error in (no error)"=w59, "Image In"=w62, "RefBrdIn"=w44) -> ("error out"=w60:errorcluster, "Image"=w61:T1, "RefBrdOut"=w43:u32)  [unwired: 6 in]
  n325 = call <vilib>:"Close.vi"("error in (no error)"=w60, "RefBrdIn"=w43) -> ("error out"=w42:errorcluster)  [unwired: 8 in, 1 out]
  n326 = call "Imaq Dispose"("Image"=w61, "error in (no error)"=w42) -> ("error out"=w24:errorcluster)  [unwired: 4 in]
  n327 = flat-sequence {
    tunnel: w24 -> [_]
    frame #0 {
      n328 = Stop(stop? (T)=TRUE ("停止？(T)")) -> ()
    }
  }
